vi "Autosize Table Columns.vi"(4 "error in (no error)":errorcluster, 6 "Options":T1={"Whitespace Border"=10, "Resize Table"=FALSE, "Number of Columns"=20, "Default Width"=50}, 7 "Table Ref":refnum<vi>) -> (0 "error out":errorcluster)   [LabVIEW 2015]
doc: "This VI resizes each column of the table specified by Table Ref based on the widest entry of the column. Additionally, if Resize Table? is TRUE, the VI will set the table width based on the number of populated columns."
panel:
  # "The original code was found in NI Discussion Forum, by ceger\nhttp://forums.ni.com/ni/board/message?board.id=170&message.id=356189\n\nThis version is modified to handle\n1)\tAutosize Row's Header column and added default width size for empty table.\n2)\tRun from JKI right-click framework"
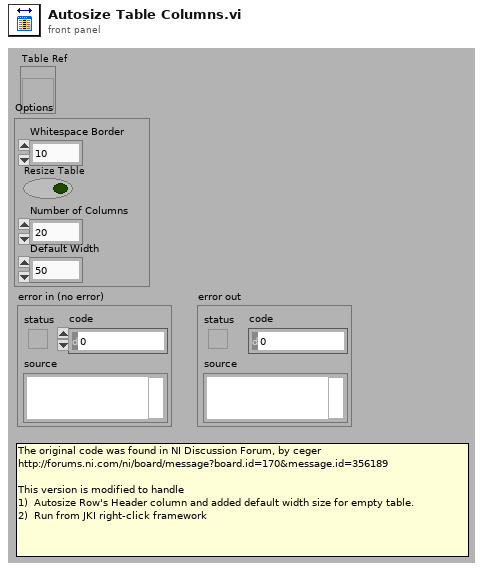
[diagram p1: front panel]
types:
  T1 = cluster{"Whitespace Border":i16, "Resize Table":bool, "Number of Columns":i32, "Default Width":u32}
  T2 = enum16{"User-specified Font", "Application Font", "System Font", "Dialog Font"}
  T3 = cluster{"Font Name:":string, "Size":i16, "Strikeout?":bool, "Italic?":bool, "Underline?":bool, "Outline?":bool, "Shadow?":bool, "Bold?":bool}
  T4 = typedef "LVRowAndColumnTypeDef.ctl" = cluster{"Row":i32, "Column":i32}
  T5 = cluster{"left":i16, "top":i16, "right":i16, "bottom":i16}
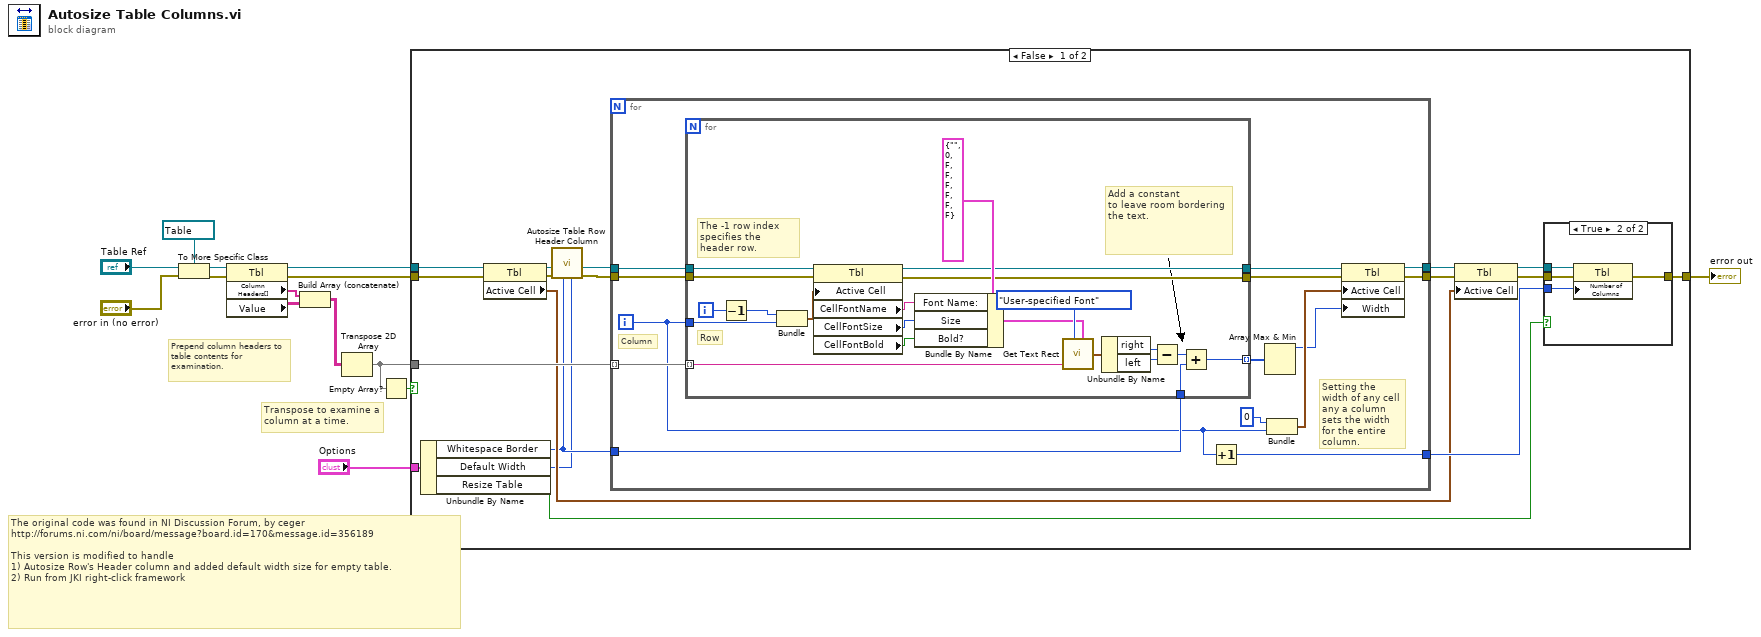
[diagram p0: block diagram]
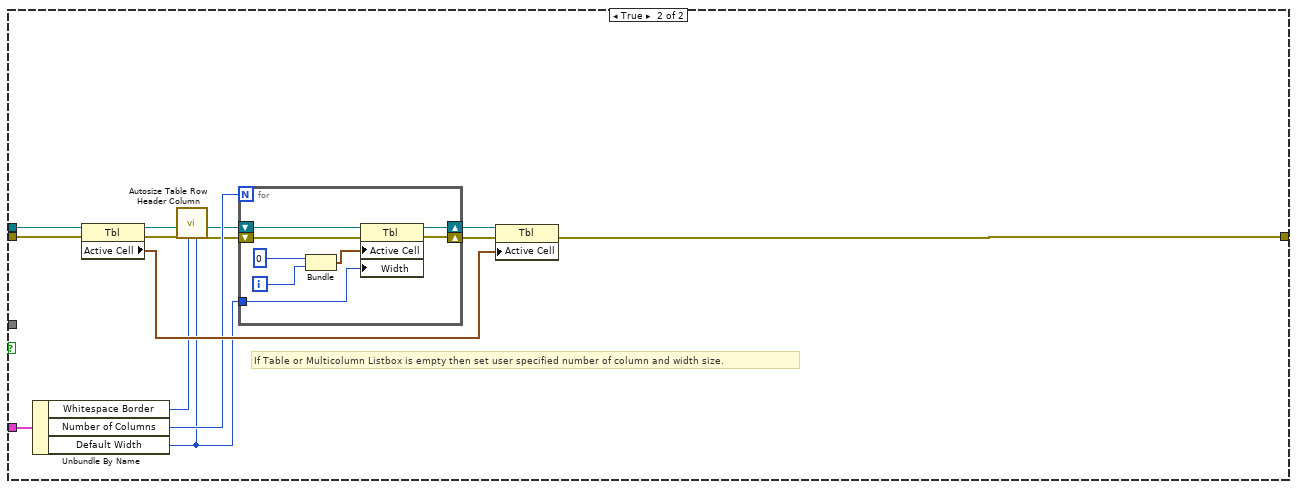
[diagram p3: hidden frame]
diagram:
  # "The original code was found in NI Discussion Forum, by ceger\nhttp://forums.ni.com/ni/board/message?board.id=170&message.id=356189\n\nThis version is modified to handle\n1)\tAutosize Row's Header column and added default width size for empty table.\n2)\tRun from JKI right-click framework"
  # "Transpose to examine a column at a time."
  # "Prepend column headers to table contents for examination."
  n1 = To More Specific Class(target class=refnum<vi> refnum ("Table Ref"), reference="Table Ref", error in="error in (no error)") -> (specific class reference=w7:refnum<vi>, error out=w5:errorcluster)
  n2 = property class="Tbl"(reference=w7, error in=w5) -> (reference out=w14:refnum<vi>, error out=w12:errorcluster, "Column Headers[]"=w2:string[], "Value"=w11:string[][])
  n3 = Build Array (concatenate)(w2, w11) -> (w13:string[][])
  n4 = Transpose 2D Array(2D array=w13) -> (transposed array=w1:string[][])
  n5 = Empty Array?(array=w1) -> (empty?=w4:bool)
  n6 = case shown="False" w4 {
    tunnel: w14 -> [w24 w83]
    tunnel: w1 -> [w32 _]
    tunnel: w12 -> [w25 w84]
    tunnel: [w30 w85] -> w10
    tunnel: "Options" -> [w22 w80]
    frame False {
      n7 = Unbundle By Name(w22) -> ("Whitespace Border"=w16:i16, "Default Width"=w15:u32, "Resize Table"=w21:bool)
      n8 = property class="Tbl"(reference=w24, error in=w25) -> (reference out=w20:refnum<vi>, error out=w18:errorcluster, "Active Cell"=w23:T4)
      n9 = call "Autosize Table Row Header Column.vi"("Default Width"=w15, "Whitespace Border"=w16, "error in"=w18, "reference in"=w20) -> ("error out"=w17:errorcluster, "reference out"=w19:refnum<vi>)  [unwired: 6 out]
      n10 = for {
        tunnel: w32 -> [w46] mode=indexing
        tunnel: w19 -> [w45]
        tunnel: w17 -> [w43]
        tunnel: [w37] -> w29
        tunnel: [w36] -> w27
        tunnel: [w35] -> w31
        tunnel: w16 -> [w34]
        i -> [w33]
        # "Setting the width of any cell any a column sets the width for the entire column."
        # "Column"
        n11 = for {
          tunnel: w46 -> [w59] mode=indexing
          tunnel: w45 -> [w67]
          tunnel: w33 -> [w66]
          tunnel: [w49] -> w44 mode=indexing
          tunnel: w43 -> [w54]
          tunnel: [w53] -> w41
          tunnel: [w52] -> w42
          tunnel: w34 -> [w47]
          i -> [w48]
          # "The -1 row index specifies the header row."
          # "Add a constant\nto leave room bordering the text."
          # "Row"
          n12 = Decrement(x=w48) -> (x-1=w55:i32)
          n13 = Bundle(w55, w66) -> (w65:cluster{i32, i32})  [unwired: 1 out]
          n14 = property class="Tbl"(reference=w67, error in=w54, "Active Cell"=w65) -> (reference out=w52:refnum<vi>, error out=w53:errorcluster, "CellFontName"=w63:string, "CellFontSize"=w50:u32, "CellFontBold"=w62:bool)
          n15 = Bundle By Name(cluster=T3 {"Font Name:"="", "Size"=0, "Strikeout?"=FALSE, "Italic?"=FALSE, "Underline?"=FALSE, "Outline?"=FALSE, "Shadow?"=FALSE, "Bold?"=FALSE} ("[user-specified font]"), "Font Name:"=w63, "Size"=w50, "Bold?"=w62) -> (w60:T3)
          n16 = call <vilib>:"Get Text Rect.vi"("desired font(Application)"=T2."User-specified Font", "text"=w59, "[user-specified font]"=w60) -> ("rect"=w58:T5)  [unwired: 3 in, 3 out]
          n17 = Unbundle By Name(w58) -> ("right"=w57:i16, "left"=w56:i16)
          n18 = Subtract(x=w57, y=w56) -> (x-y=w51:i16)
          n19 = Add(x=w51, y=w47) -> (x+y=w49:i16)
        }
        n20 = Increment(x=w33) -> (x+1=w35:i32)
        n21 = Array Max & Min(array=w44) -> (max value=w38:i16)  [unwired: 3 out]
        n22 = Bundle(0, w33) -> (w39:cluster{i32, i32})  [unwired: 1 out]
        n23 = property class="Tbl"(reference=w42, error in=w41, "Active Cell"=w39, "Width"=w38) -> (reference out=w36:refnum<vi>, error out=w37:errorcluster)
      }
      n24 = property class="Tbl"(reference=w27, error in=w29, "Active Cell"=w23) -> (reference out=w28:refnum<vi>, error out=w26:errorcluster)
      n25 = case shown="True" w21 {
        tunnel: w28 -> [_ w72]
        tunnel: w26 -> [w68 w71]
        tunnel: w31 -> [_ w70]
        tunnel: [w68 w69] -> w30
        frame False {
        }
        frame True {
          n26 = property class="Tbl"(reference=w72, error in=w71, "Number of Columns"=w70) -> (error out=w69:errorcluster)  [unwired: 1 out]
        }
      }
    }
    frame True {
      # "If Table or Multicolumn Listbox is empty then set user specified number of column and width size."
      n27 = Unbundle By Name(w80) -> ("Whitespace Border"=w73:i16, "Number of Columns"=w79:i32, "Default Width"=w74:u32)
      n28 = property class="Tbl"(reference=w83, error in=w84) -> (reference out=w78:refnum<vi>, error out=w76:errorcluster, "Active Cell"=w81:T4)
      n29 = call "Autosize Table Row Header Column.vi"("Default Width"=w74, "Whitespace Border"=w73, "error in"=w76, "reference in"=w78) -> ("error out"=w75:errorcluster, "reference out"=w77:refnum<vi>)  [unwired: 6 out]
      n30 = for {
        N: w79 -> [_]
        shift-right: [w93] -> w86
        shift-left: w75 -> [w94]
        shift-right: [w89] -> w82
        shift-left: w77 -> [w90]
        tunnel: w74 -> [w88]
        i -> [w87]
        n31 = Bundle(0, w87) -> (w91:cluster{i32, i32})  [unwired: 1 out]
        n32 = property class="Tbl"(reference=w90, error in=w94, "Active Cell"=w91, "Width"=w88) -> (reference out=w89:refnum<vi>, error out=w93:errorcluster)
      }
      n33 = property class="Tbl"(reference=w82, error in=w86, "Active Cell"=w81) -> (error out=w85:errorcluster)  [unwired: 1 out]
    }
  }
  "error out" <- w10
